vi "NI VeriStand - Set Alarm Acknowledgement Status.vi"(8 "error in (no error)":errorcluster, 10 "Status":T1, 11 "Alarm in":T2) -> (0 "error out":errorcluster, 3 "Alarm out":T2)   [LabVIEW 2020, in "NI_VS Alarm ExecutionAPI.lvlib"]
doc: "Sets whether an alarm is acknowledged or unacknowledged. You can optionally configure alarms to require acknowledgement before VeriStand resets the alarm."
uses:
  <vilib>/NI VeriStand/Execution/Alarm/NI_VS Alarm ExecutionAPI.lvlib
  <vilib>/NI VeriStand/Execution/Alarm/AlarmAPI.ctl
  NationalInstruments.VeriStand.ClientAPI
  <vilib>/NI VeriStand/Execution/Alarm/AcknowledgementStatus.ctl
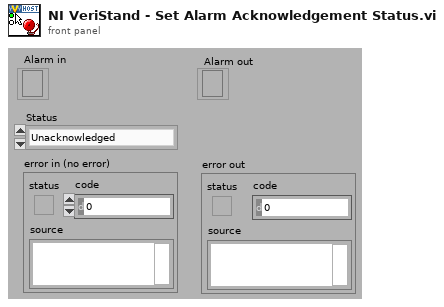
[diagram p1: front panel]
types:
  T1 = typedef "NI_VS Alarm ExecutionAPI.lvlib/AcknowledgementStatus.ctl" = enum16{"Unacknowledged", "Acknowledged"}
  T2 = typedef "NI_VS Alarm ExecutionAPI.lvlib/AlarmAPI.ctl" = refnum<k24>
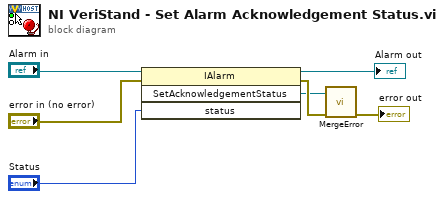
[diagram p0: block diagram]
diagram:
  n1 = invoke class="IAlarm" method="SetAcknowledgementStatus"(reference="Alarm in", error in="error in (no error)", "status"="Status") -> (reference out=→"Alarm out":T2, error out=w7:errorcluster, "SetAcknowledgementStatus"=w4:refnum<k24>)  [unwired: 1 in, 1 out]
  n2 = call <vilib>:"MergeError.vi"("error in (no error)"=w7, "Error"=w4) -> ("error out"=→"error out":errorcluster)  [unwired: 9 out]
